vi "Obtain Transfer Group.vi"(8 "error in (no error)":errorcluster, 10 "command parameters":T1, 11 "Transceiver Thread in":refnum<class "Transceiver Thread.lvclass">) -> (0 "error out":errorcluster, 2 "Transfer Group":refnum<class "Transfer Group.lvclass">, 3 "Transceiver Thread out":refnum<class "Transceiver Thread.lvclass">)   [LabVIEW 2017, in "Data Sharing Framework Core.lvlib" / "Data Sharing Framework Engine.lvlib" / "Transceiver Thread.lvclass"]
uses:
  Transceiver Thread.lvclass
  Interfaces/Transceiver Interface/Command Parameters.ctl
  Transfer Group/Transfer Group.lvclass
  Transceiver Thread.lvclass/Transceiver Thread.ctl
  Transfer Group/Transfer Group.lvclass/Transfer Group.ctl
  Timing/Engine Timing.lvclass/Engine Timing.ctl
  Get Transfer Group.vi
  Transfer Group/Get Timing.vi
  Timing/Set Iteration Count.vi
  Transfer Group/Set Timing.vi
  Timing/Set Iteration.vi
  Interfaces/Transceiver Interface/Transceiver Interface.lvclass
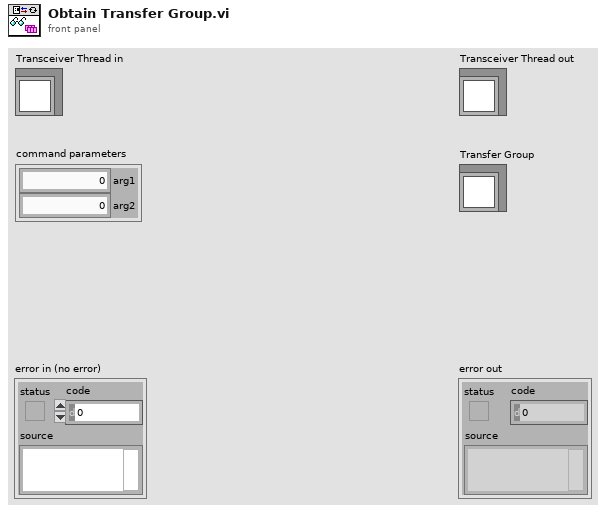
[diagram p1: front panel]
types:
  T1 = typedef "Data Sharing Framework Core.lvlib/Data Sharing Framework Engine.lvlib/Transceiver Interface.lvclass/Command Parameters.ctl" = cluster{"arg1":u64, "arg2":u64}
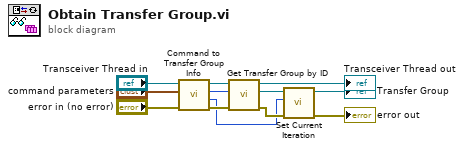
[diagram p0: block diagram]
diagram:
  n1 = call "Command to Transfer Group Info.vi"("error in (no error)"="error in (no error)", "command parameters"="command parameters", "Transceiver Thread in"="Transceiver Thread in") -> ("error out"=w10:errorcluster, "Transfer Group iteration"=w2:u64, "Transfer Group id"=w11:i32, "Transceiver Thread out"=w12:refnum<class "Transceiver Thread.lvclass">)  [unwired: 5 in]
  n2 = call "Get Transfer Group by ID.vi"("error in (no error)"=w10, "Transfer Group id"=w11, "Transceiver Thread in"=w12) -> ("error out"=w5:errorcluster, "Transfer Group"=w6:refnum<class "Transfer Group.lvclass">, "Transceiver Thread out"=→"Transceiver Thread out":refnum<class "Transceiver Thread.lvclass">)  [unwired: 6 in]
  n3 = call "Set Current Iteration.vi"("error in (no error)"=w5, "iteration"=w2, "Transfer Group in"=w6) -> ("error out"=→"error out":errorcluster, "Transfer Group out"=→"Transfer Group":refnum<class "Transfer Group.lvclass">)  [unwired: 7 in]
